vi "Set EM Gain.vi"(8 "error in (no error)":errorcluster, 11 "CCDCamera in":refnum<class "Ixon_Ultra.lvclass">) -> (0 "error out":errorcluster, 3 "CCDCamera out":refnum<class "Ixon_Ultra.lvclass">)   [LabVIEW 2018, in "Ixon_Ultra.lvclass"]
doc: "Set EM gain"
uses:
  Ixon_Ultra.lvclass
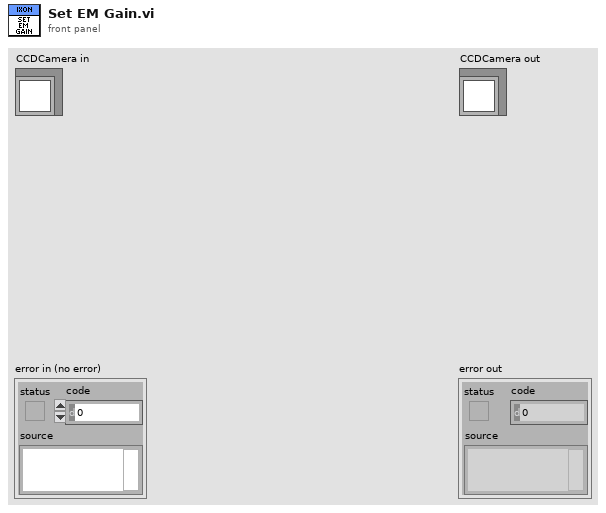
[diagram p1: front panel]
types:
  T1 = cluster{"EM_MODE":u16, "EM_GAIN":u16, "FRAME_TRANSFER":bool}
  T2 = cluster{"PREAMP":u16, "READOUT_RATE":u16, "VERTICAL_SHIFT_SPEED":u16, "READ_MODE":u16, "VERTICAL_CLOCK_VOLTAGE":u16, "ACQUISITION_MODE":u16, "AD_CHANNEL":u16, "SHUTTER_TTL":u16, "SHUTTER_OPENING_TIME":u16, "SHUTTER_CLOSING_TIME":u16, "SHUTTER_MODE":u16, "TRIGGER_MODE":u16, "VBIN":u16, "INITIAL_LINE":u16, "INITIAL_COLUMN":u16, "FINAL_LINE":u16, "FINAL_COLUMN":u16, "HBIN":u16, "TEMP":i32, "COOLER_POWER_STATUS":u16}
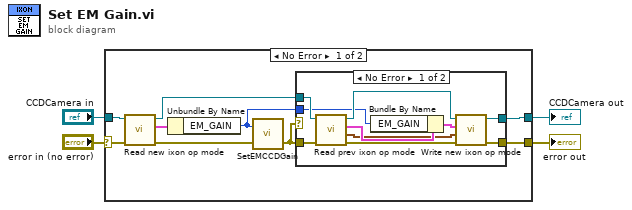
[diagram p0: block diagram]
diagram:
  n1 = case shown="No Error" "error in (no error)" {
    selector: "error in (no error)" -> [w9 w27]
    tunnel: [w12 w27] -> w4
    tunnel: [w6 w26] -> w3
    tunnel: "CCDCamera in" -> [w8 w26]
    frame No Error {
      n2 = call-dynamic "Read new ixon op mode.vi"("error in (no error)"=w9, "Sim_Ixon_Ultra in"=w8) -> ("error out"=w10:errorcluster, "new ixon op mode"=w11:T1, "Sim_Ixon_Ultra out"=w7:refnum<class "Ixon_Ultra.lvclass">)  [unwired: 6 in, 1 out]
      n3 = Unbundle By Name(w11) -> ("EM_GAIN"=w5:u16)
      n4 = call <userlib>:"SetEMCCDGain.vi"("error in (no error)"=w10, "gain"=w5) -> ("error out"=w13:errorcluster)  [unwired: 1 out]
      n5 = case shown="No Error" w13 {
        tunnel: [w16 w25] -> w12
        tunnel: w13 -> [w17 w25]
        tunnel: w7 -> [w23 w24]
        tunnel: [w15 w24] -> w6
        tunnel: w5 -> [w14 _]
        frame No Error {
          n6 = call-dynamic "Read prev ixon op mode.vi"("error in (no error)"=w17, "Sim_Ixon_Ultra in"=w23) -> ("error out"=w18:errorcluster, "prev operation mode"=w19:T2, "prev ixon op mode"=w22:T1, "Sim_Ixon_Ultra out"=w20:refnum<class "Ixon_Ultra.lvclass">)  [unwired: 6 in]
          n7 = Bundle By Name(cluster=w22, "EM_GAIN"=w14) -> (w21:T1)
          n8 = call-dynamic "Write new ixon op mode.vi"("error in (no error)"=w18, "new operation mode"=w19, "new ixon op mode"=w21, "Sim_Ixon_Ultra in"=w20) -> ("error out"=w16:errorcluster, "Sim_Ixon_Ultra out"=w15:refnum<class "Ixon_Ultra.lvclass">)  [unwired: 6 in]
        }
        frame Error {
        }
      }
    }
    frame Error {
    }
  }
  "error out" <- w4
  "CCDCamera out" <- w3
